vi "AutoSelector.vi"(8 "3":bool, 9 "2":bool, 10 "1":bool, 11 "0":bool) -> (3 "Auto":i32)   [LabVIEW 2014]
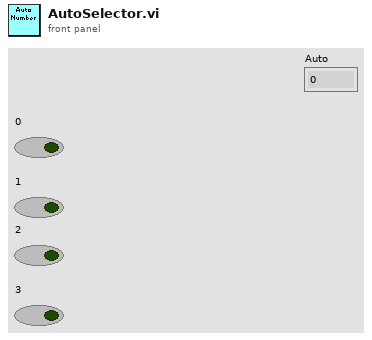
[diagram p1: front panel]
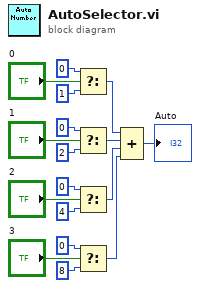
[diagram p0: block diagram]
diagram:
  n1 = Select(t=0, s="0", f=1) -> (s? t:f=w5:i32)
  n2 = Select(t=0, s="1", f=2) -> (s? t:f=w4:i32)
  n3 = Select(t=0, s="2", f=4) -> (s? t:f=w3:i32)
  n4 = Select(t=0, s="3", f=8) -> (s? t:f=w2:i32)
  n5 = Compound Arithmetic op=ADD(w5, w4, w3, w2) -> (→"Auto":i32)
